vi "SMO.Basic--Process.vi"(8 "error in (no error)":errorcluster, 11 "SMO.Basic in":refnum<class "SMO.Basic.lvclass">) -> (0 "error out":errorcluster)   [LabVIEW 2013, in "SMO.Basic.lvclass"]
uses:
  SMO.Basic.lvclass
  <vilib>/JKI/JKI SMO/SMO/SMO.lvclass
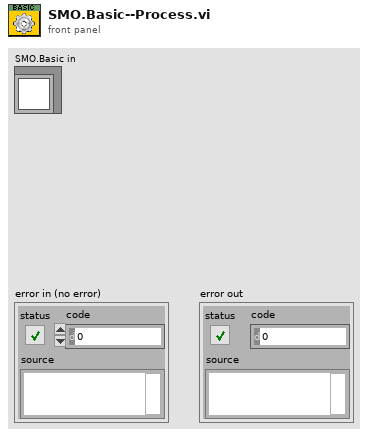
[diagram p1: front panel]
types:
  T1 = enum32{"invalid app kind", "Development System", "Run Time System", "Student Edition", "Embedded LabVIEW", "Evaluation", "Custom"}
  T2 = cluster{"Current VI Reference":refnum<vi>, "Close Panel on Exit?":bool, "error":errorcluster, "Standalone":bool}
  T3 = enum32{"Invalid", "Standard", "Closed", "Hidden", "Minimized", "Maximized"}
  T4 = typedef "SMO.lvclass/SMOState --Enum.ctl" = enum16{"unknown", "Created", "Started", "Stopped"}
  T5 = cluster{"Core":cluster{"Current VI Reference":refnum<vi>, "Close Panel on Exit?":bool, "error":errorcluster, "Standalone":bool}, "Self Reference":refnum<class "SMO.Basic.lvclass">, "Your string data":string}
  T6 = typedef "SMO.lvclass/Protected Events.ctl" = cluster{"StopProcesses":refnum<user-event>, "AbortProcesses":refnum<user-event>, "Config Changed":refnum<user-event>}
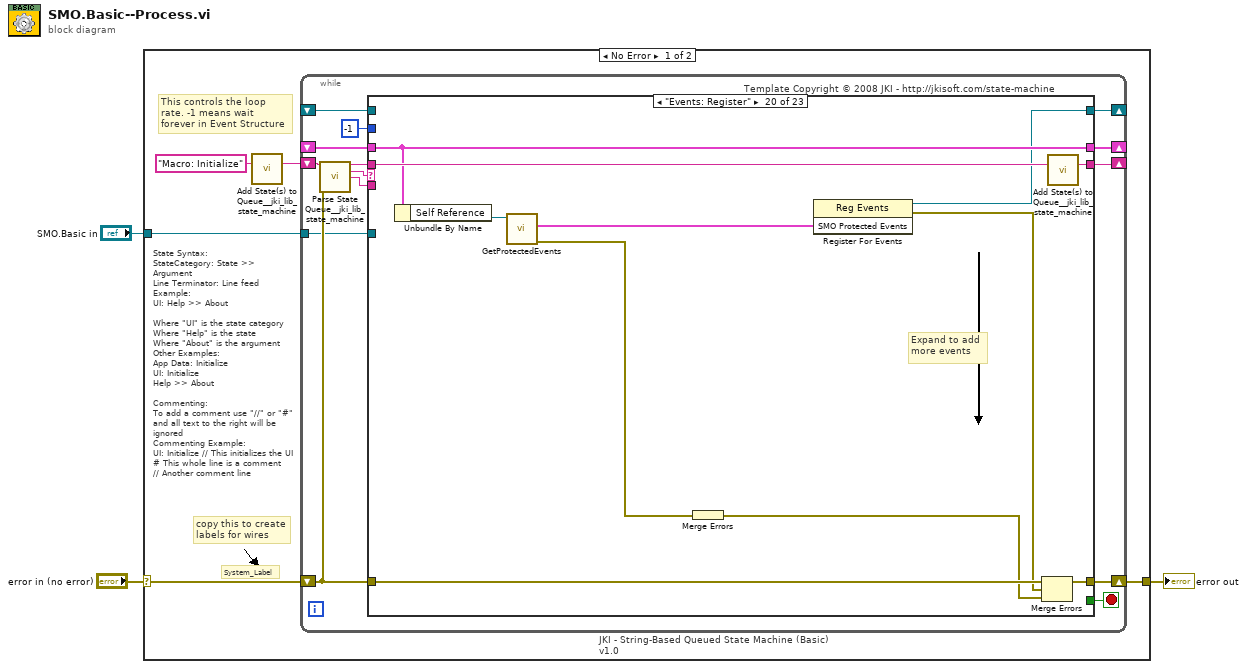
[diagram p0: block diagram]
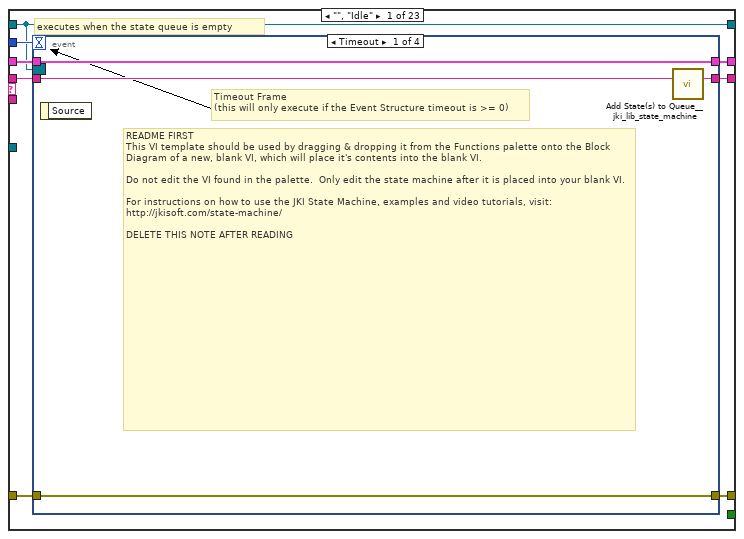
[diagram p2: hidden frame]
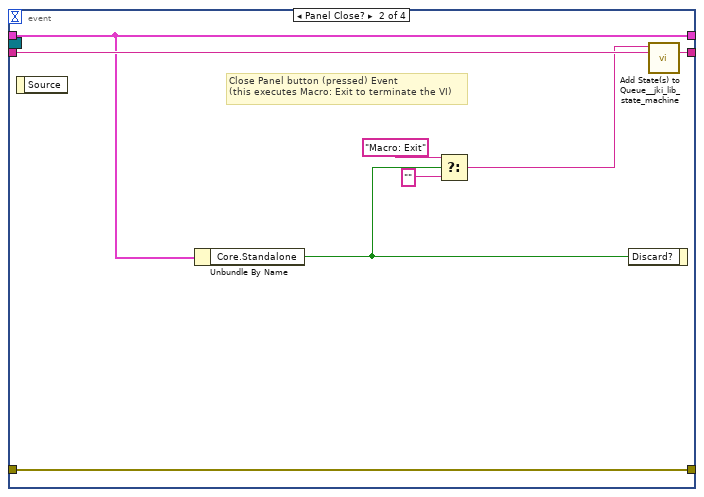
[diagram p3: hidden frame]
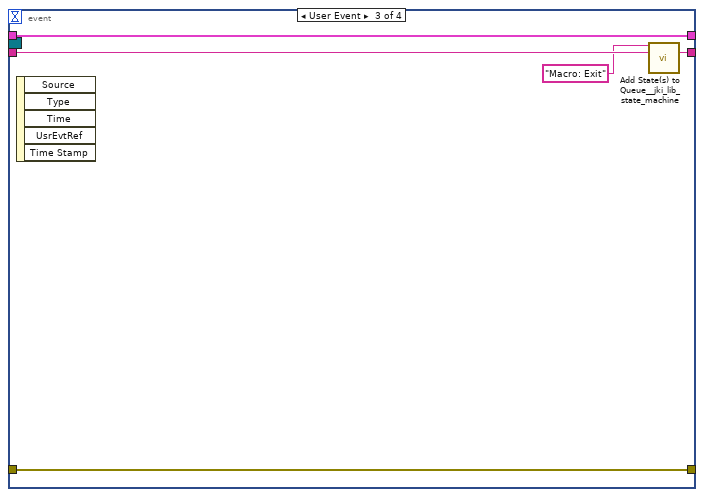
[diagram p4: hidden frame]
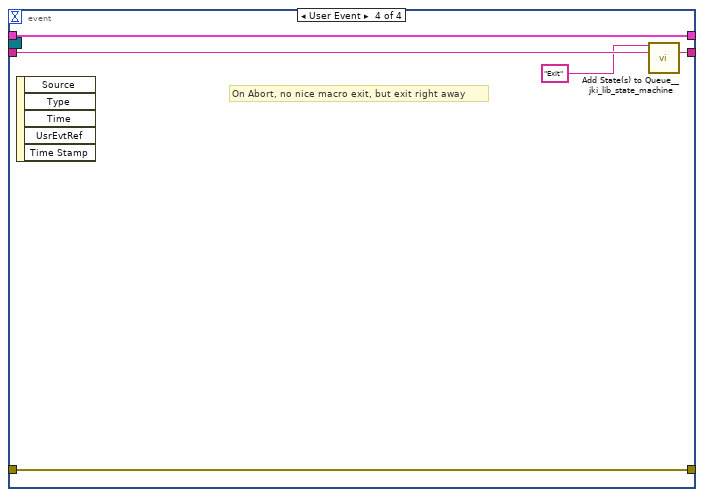
[diagram p5: hidden frame]
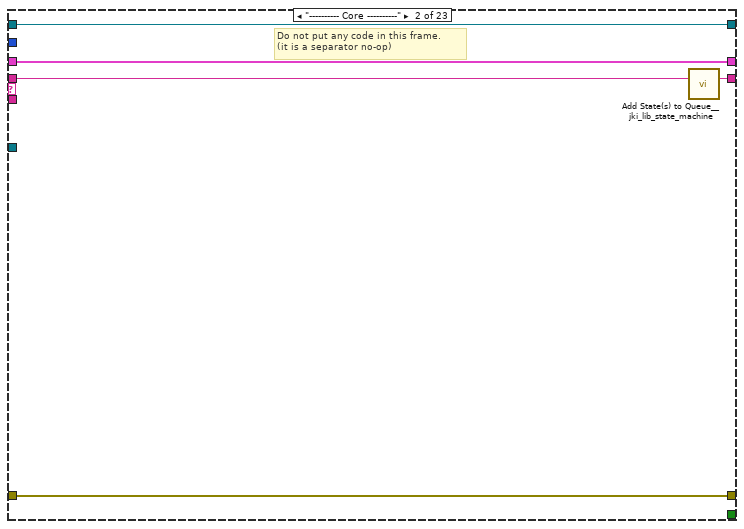
[diagram p6: hidden frame]
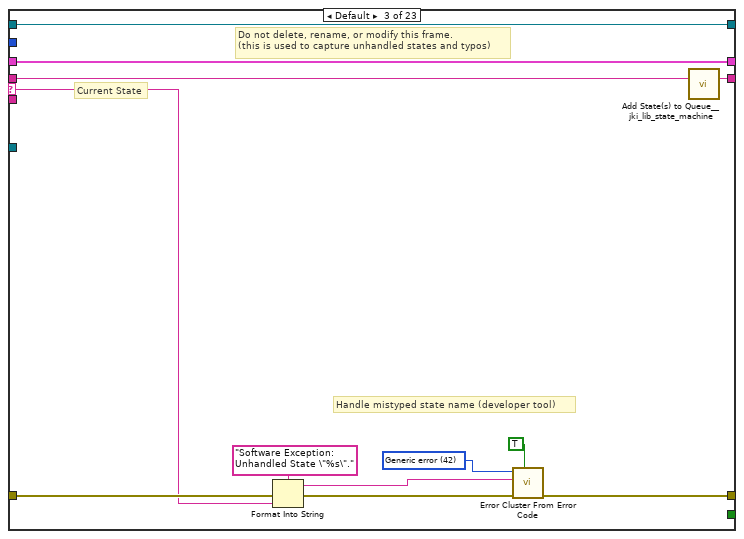
[diagram p7: hidden frame]
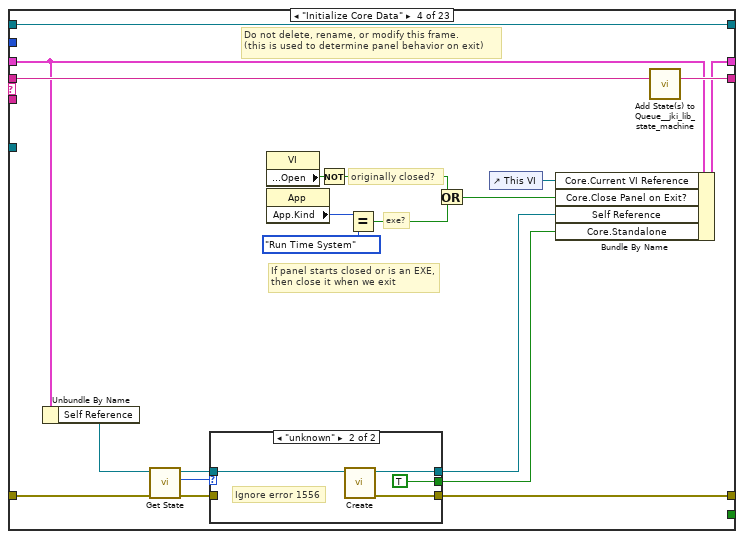
[diagram p8: hidden frame]
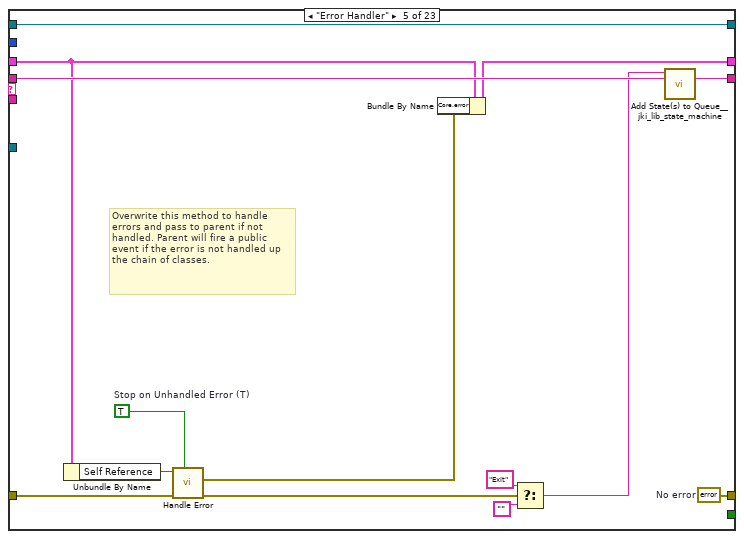
[diagram p10: hidden frame]
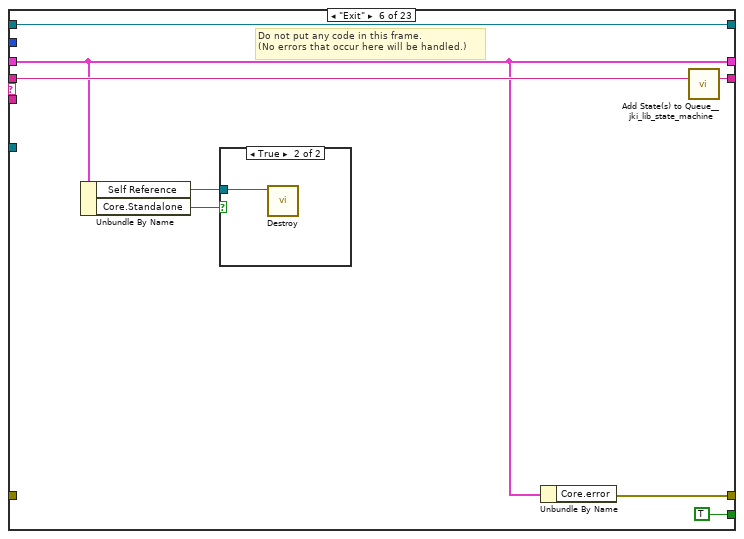
[diagram p11: hidden frame]
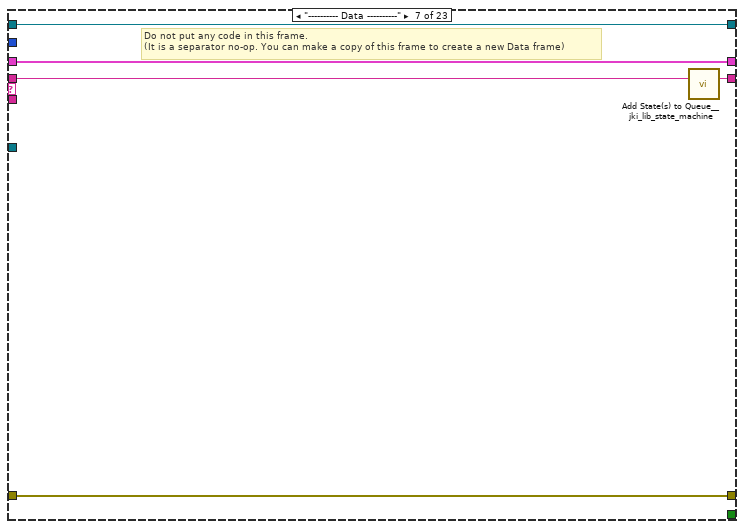
[diagram p13: hidden frame]
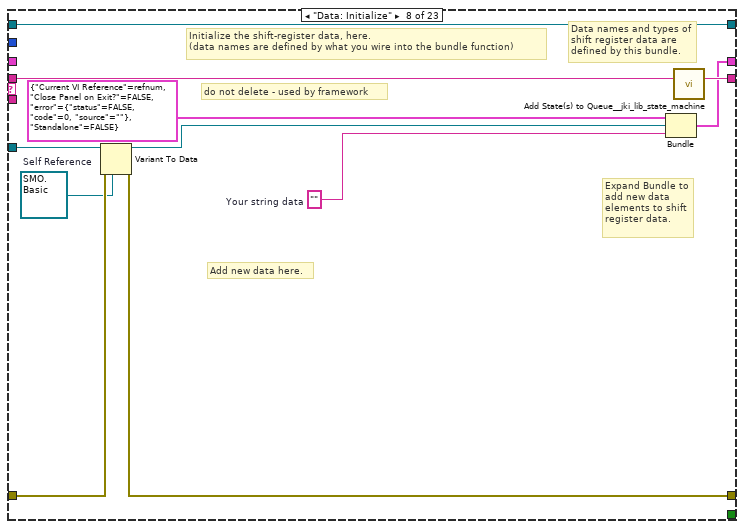
[diagram p14: hidden frame]
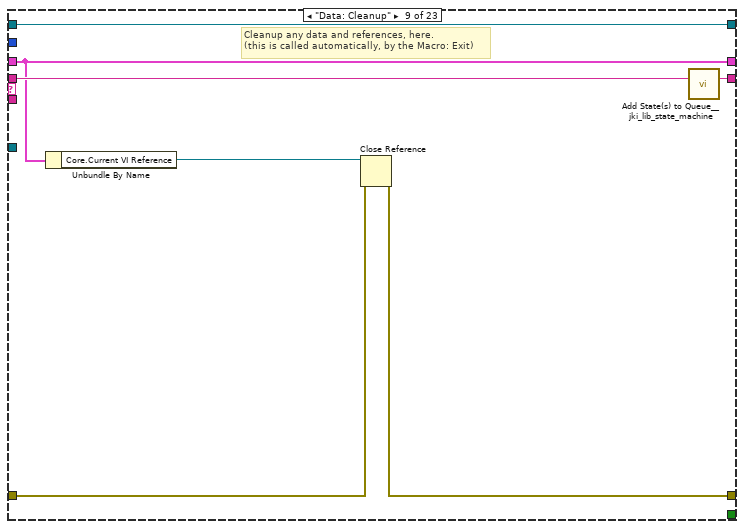
[diagram p15: hidden frame]
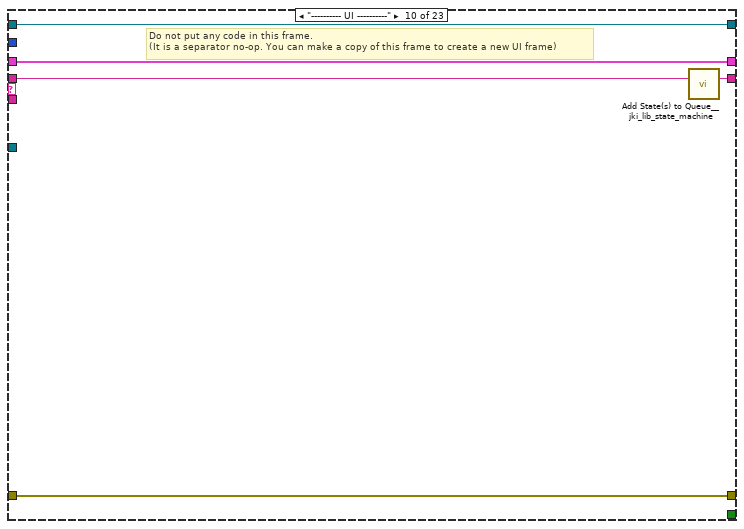
[diagram p16: hidden frame]
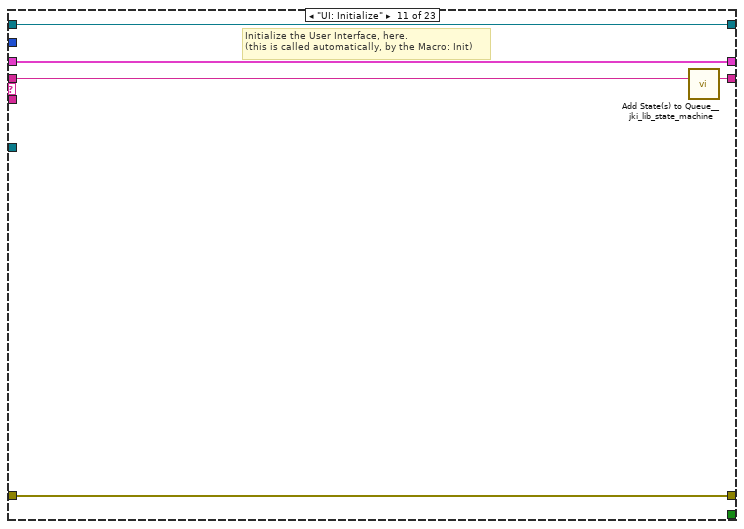
[diagram p17: hidden frame]
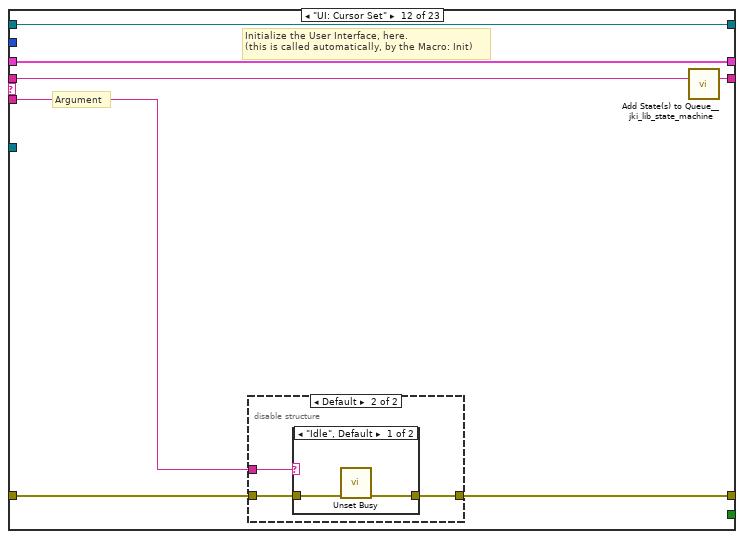
[diagram p18: hidden frame]
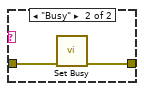
[diagram p20: hidden frame]
diagram:
  n1 = case shown="No Error" "error in (no error)" {
    selector: "error in (no error)" -> [w5 w280]
    tunnel: "SMO.Basic in" -> [w6 _]
    tunnel: [w4 w280] -> w3
    frame No Error {
      # "State Syntax:\nStateCategory: State >> Argument\nLine Terminator: Line feed\nExample:\nUI: Help >> About\n\nWhere \"UI\" is the state category\nWhere \"Help\" is the state\nWhere \"About\" is the argument\nOther Examples:\nApp Data: Initialize\nUI: Initialize\nHelp >> About\n\nCommenting:\nTo add a comment use \"//\" or \"#\" and all text to the right will be ignored\nCommenting Example:\nUI: Initialize // This initializes the UI\n# This whole line is a comment\n// Another comment line"
      # "copy this to create labels for wires"
      # "This controls the loop rate. -1 means wait forever in Event Structure"
      # "System_Label"
      n2 = call <vilib>:"Add State(s) to Queue__jki_lib_state_machine.vi"("State(s) in (\"\")"="Macro: Initialize") -> ("States Out"=w8:string)  [unwired: 14 in]
      n3 = while "JKI - String-Based Queued State Machine (Basic) v1.0" {
        shift-right: [w15] -> _
        shift-left: _ -> [w14]
        shift-right: [w18] -> w4
        shift-left: w5 -> [w12]
        shift-right: [w17] -> _
        shift-left: w8 -> [w19]
        tunnel: w6 -> [w11]
        shift-right: [w10] -> _
        shift-left: _ -> [w9]
        stop <- w16 stop-if-true
        # "Template Copyright © 2008 JKI - http://jkisoft.com/state-machine"
        n4 = call <vilib>:"Parse State Queue__jki_lib_state_machine.vi"("State Queue"=w19, "Error In (no error)"=w12) -> ("Remaining States"=w21:string, "Current State"=w22:string, "Arguments"=w20:string)  [unwired: 11 in]
        n5 = case shown="\"Events: Register\"" w22 {
          selector: w22 -> [_ _ w59 _ _ _ _ _ _ _ _ _ _ _ _ _ _ _ _ _ _ _ _]
          tunnel: w21 -> [w30 w57 w63 w89 w109 w117 w123 w134 w141 w146 w151 w158 w174 w206 w212 w223 w228 w237 w250 w261 w267 w272 w279]
          tunnel: w20 -> [_ _ _ _ _ _ _ _ _ _ _ w152 w168 _ _ _ _ _ _ _ _ _ _]
          tunnel: w14 -> [w28 w54 w61 w78 w103 w112 w120 _ w136 w143 w149 w156 w170 w203 w208 w214 w225 w234 w247 w259 w265 w270 w275]
          tunnel: [w27 w55 w65 w73 w104 w113 w121 w129 w137 w144 w148 w153 w171 w204 w210 w221 w226 w231 w248 w254 w263 w268 w276] -> w18
          tunnel: w12 -> [w26 w55 w64 w77 w105 _ w121 w130 w138 w144 w148 w154 w172 w204 w210 w221 w226 w232 w248 w255 w263 w268 w276]
          tunnel: [w29 w56 w62 w88 w108 w116 w122 w133 w140 w145 w150 w157 w173 w205 w211 w222 w227 w236 w249 w260 w266 w271 w278] -> w17
          tunnel: [_ _ _ _ _ TRUE _ _ _ _ _ _ _ _ _ _ _ _ _ _ _ _ _] -> w16
          tunnel: [w25 w54 w61 w87 w102 w112 w120 w132 w136 w143 w149 w156 w170 w203 w208 w214 w225 w234 w247 w259 w265 w270 w274] -> w15
          tunnel: -1 ("Timeout") -> [w24 _ _ _ _ _ _ _ _ _ _ _ _ _ _ _ _ _ _ _ _ _ _]
          tunnel: w11 -> [_ _ _ _ _ _ _ w127 _ _ _ _ _ _ _ _ _ _ _ _ _ _ _]
          tunnel: [w23 w53 w58 w80 w107 w114 w119 w125 w135 w142 w147 w155 w167 w202 w209 w215 w224 w235 w246 w258 w264 w269 w277] -> w10
          tunnel: w9 -> [w23 w53 w58 w80 w107 w114 w119 w125 w135 w142 w147 w155 w167 w202 w209 w215 w224 w235 w246 _ w264 w269 w277]
          frame "", "Idle" {
            # "executes when the state queue is empty"
            n6 = event shown="[0] Timeout" {
              selector: w23 -> [_ _ _ _]
              dyn-events: _ -> [_ _ _ _]
              timeout: w24 -> [_ _ _ _]
              tunnel: w30 -> [w34 w42 w47 w52]
              tunnel: [w33 w41 w46 w51] -> w29
              tunnel: w28 -> [w32 w39 w44 w49]
              tunnel: [w31 w40 w45 w50] -> w27
              tunnel: w26 -> [w31 w40 w45 w50]
              tunnel: [w32 w39 w44 w49] -> w25
              event Timeout {
                # "README FIRST\nThis VI template should be used by dragging & dropping it from the Functions palette onto the Block Diagram of a new, blank VI, which will place it's contents into the blank VI.\n\nDo not edit the VI found in the palette.  Only edit the state machine after it is placed into your blank VI.\n\nFor instructions on how to use the JKI State Machine, examples and video tutorials, visit:\nhttp://jkisoft.com/state-machine/\n\nDELETE THIS NOTE AFTER READING"
                # "Timeout Frame\n(this will only execute if the Event Structure timeout is >= 0)"
                n7 = event-data() -> ()  [unwired: 1 in, 1 out]
                n8 = call <vilib>:"Add State(s) to Queue__jki_lib_state_machine.vi"("State(s) in (\"\")"=w34) -> ("States Out"=w33:string)  [unwired: 14 in]
              }
              event Panel Close? {
                # "Close Panel button (pressed) Event\n(this executes Macro: Exit to terminate the VI)"
                n9 = event-data() -> ()  [unwired: 1 in, 1 out]
                n10 = Unbundle By Name(w39) -> ("Core.Standalone"=w38:bool)
                n11 = Select(t="Macro: Exit", s=w38, f="") -> (s? t:f=w35:string)
                n12 = event-data("Discard?"=w38) -> ()  [unwired: 1 in, 1 out]
                n13 = call <vilib>:"Add State(s) to Queue__jki_lib_state_machine.vi"("State(s) in Front (\"\")"=w35, "State(s) in (\"\")"=w42) -> ("States Out"=w41:string)  [unwired: 13 in]
              }
              event User Event {
                n14 = event-data() -> ()  [unwired: 1 in, 5 out]
                n15 = call <vilib>:"Add State(s) to Queue__jki_lib_state_machine.vi"("State(s) in Front (\"\")"="Macro: Exit", "State(s) in (\"\")"=w47) -> ("States Out"=w46:string)  [unwired: 13 in]
              }
              event User Event {
                # "On Abort, no nice macro exit, but exit right away"
                n16 = event-data() -> ()  [unwired: 1 in, 5 out]
                n17 = call <vilib>:"Add State(s) to Queue__jki_lib_state_machine.vi"("State(s) in Front (\"\")"="Exit", "State(s) in (\"\")"=w52) -> ("States Out"=w51:string)  [unwired: 13 in]
              }
            }
          }
          frame "---------- Core ----------" {
            # "Do not put any code in this frame.\n(it is a separator no-op)"
            n18 = call <vilib>:"Add State(s) to Queue__jki_lib_state_machine.vi"("State(s) in (\"\")"=w57) -> ("States Out"=w56:string)  [unwired: 14 in]
          }
          frame Default {
            w68 = 42 items=["No error", "Argument error", "Memory is full", "Out of zone", "End of file", "File already open", "Generic file I/O error", "File not found", "File permission error", "Disk is full", "Duplicate path", "Too many files open", "System feature not enabled", "Resource file not found", "Cannot add resource", "Resource not found", "Image not found", "Image memory error", "Pen does not exist", "Config type invalid", "Config token not found", "Config parse error", "Config memory error", "Bad external code format", "Bad external code offset", "External code not present", "Null window", "Destroy window error", "Null menu", "Print aborted", "Bad print record", "Print driver error", "Windows error during printing", "Memory error during printing", "Print dialog error", "Generic print error", "Invalid device refnum", "Device not found", "Device parameter error", "Device unit error", "Cannot open device", "Device call aborted", "Generic error", "Cancelled by user", "Object ID too low", "Object ID too high", "Object not in heap", "Unknown heap", "Unknown object (invalid DefProc)", "Unknown object (DefProc not in table)", "Message out of range", "Invalid (null) method", "Unknown message", "Manager call not supported", "Bad address", "Network operation in progress", "Network operation timed out", "Connection is busy", "Network attribute not supported", "Network error", "Address in use", "System out of memory", "Connection aborted", "Connection refused", "Not connected", "Already connected", "Connection closed", "Initialization error (interapplication manager)", "Bad occurrence", "Wait on unbound occurrence handler", "Occurrence queue overflow", "Datalog type conflict", "Unused", "Unrecognized type (interapplication manager)", "Memory corrupt", "Failed to make temporary DLL", "Old CIN version", "Drag socket not found", "Failed to load drop-object", "Failed to register OLE object", "Failed to release OLE object", "Format specifier type mismatch", "Unknown format specifier", "Too few format specifiers", "Too many format specifiers", "Scan failed", "Newer CIN version", "Error converting to variant", "Runtime menu error", "Password tampered", "Variant attribute not found", "Incompatible variant data type", "Event data is not available", "Event Store is not present", "Occurrence is not found", "Event Queue is not created", "Event info is not available", "Refnum passed is NULL", "Error retrieving Class GUID", "Error retrieving CoClass GUID", "Error retrieving TypeLib GUID.", "Bad built application magic bytes.", "Specific driver is different from the specific driver associated with the Logical Name.", "There is no session opened to the class driver.", "Max Error", "MAX - Error with config objects", "MAX - Error loading configuration", "MAX - Group not supported"]
            # "Current State"
            # "Do not delete, rename, or modify this frame.\n(this is used to capture unhandled states and typos)"
            # "Handle mistyped state name (developer tool)"
            n19 = Format Into String(format string="Software Exception: Unhandled State \"%s\"." ("message"), error in=w64, w59) -> (resulting string=w67:string, error out=w66:errorcluster)  [unwired: 1 in]
            n20 = call <vilib>:"Error Cluster From Error Code.vi"("show call chain? (False)"=TRUE, "error in (no error)"=w66, "error message (\"\")"=w67, "error code (0)"=w68) -> ("error out"=w65:errorcluster)  [unwired: 5 in]
            n21 = call <vilib>:"Add State(s) to Queue__jki_lib_state_machine.vi"("State(s) in (\"\")"=w63) -> ("States Out"=w62:string)  [unwired: 14 in]
          }
          frame "Initialize Core Data" {
            # "Do not delete, rename, or modify this frame.\n(this is used to determine panel behavior on exit)"
            # "originally closed?"
            # "exe?"
            # "If panel starts closed or is an EXE, then close it when we exit"
            n22 = Unbundle By Name(w78) -> ("Self Reference"=w76:refnum<class "SMO.Basic.lvclass">)
            n23 = call <vilib>:"Get State.vi"("error in (no error)"=w77, "SMO"=w76) -> ("error out"=w74:errorcluster, "SMO State"=w70:T4, "SMO out"=w75:refnum<class "SMO.Basic.lvclass">)  [unwired: 7 in]
            n24 = case shown="\"unknown\"" w70 {
              tunnel: w75 -> [w91 w95]
              tunnel: w74 -> [w90 _]
              tunnel: [w90 w94] -> w73
              tunnel: [w91 w93] -> w72
              tunnel: [_ TRUE] -> w71
              frame Default {
              }
              frame "unknown" {
                # "Ignore error 1556"
                n25 = call <vilib>:"Create.vi"("SMO"=w95) -> ("error out"=w94:errorcluster, "SMO out"=w93:refnum<class "SMO.Basic.lvclass">)  [unwired: 8 in, 1 out]
              }
            }
            n26 = property class="VI"() -> ("Front Panel.Open"=w86:bool)  [unwired: 2 in, 2 out]
            n27 = property class="App"() -> ("App.Kind"=w85:T1)  [unwired: 2 in, 2 out]
            n28 = Not(x=w86) -> (.not. x?=w83:bool)
            n29 = Equal?(x=w85, y=T1."Run Time System" ("Application:Kind")) -> (x = y?=w82:bool)
            n30 = Or(x=w83, y=w82) -> (x .or. y?=w81:bool)
            n31 = control-ref of="This VI"() -> (w79:refnum<vi>)
            n32 = Bundle By Name(cluster=w78, "Core.Current VI Reference"=w79, "Core.Close Panel on Exit?"=w81, "Self Reference"=w72, "Core.Standalone"=w71) -> (w87:T5)
            n33 = call <vilib>:"Add State(s) to Queue__jki_lib_state_machine.vi"("State(s) in (\"\")"=w89) -> ("States Out"=w88:string)  [unwired: 14 in]
          }
          frame "Error Handler" {
            w96 = TRUE  # Stop on Unhandled Error (T)
            w104 = errorcluster {"status"=FALSE, "code"=0, "source"=""}  # No error
            # "Overwrite this method to handle errors and pass to parent if not handled. Parent will fire a public event if the error is not handled up the chain of classes."
            n34 = Unbundle By Name(w103) -> ("Self Reference"=w106:refnum<class "SMO.Basic.lvclass">)
            n35 = call-dynamic "Handle Error.vi"("Stop on Unhandled Error (T)"=w96, "error in"=w105, "SMO"=w106) -> ("handling error"=w97:errorcluster, "Unhandled error"=w100:errorcluster)  [unwired: 6 in, 1 out]
            n36 = Bundle By Name(cluster=w103, "Core.error"=w100) -> (w102:T5)
            n37 = Select(t="Exit", s=w97, f="") -> (s? t:f=w101:string)
            n38 = call <vilib>:"Add State(s) to Queue__jki_lib_state_machine.vi"("State(s) in Front (\"\")"=w101, "State(s) in (\"\")"=w109) -> ("States Out"=w108:string)  [unwired: 13 in]
          }
          frame "Exit" {
            # "Do not put any code in this frame.\n(No errors that occur here will be handled.)"
            n39 = Unbundle By Name(w112) -> ("Self Reference"=w111:refnum<class "SMO.Basic.lvclass">, "Core.Standalone"=w110:bool)
            n40 = case shown="True" w110 {
              tunnel: w111 -> [_ w118]
              frame False {
              }
              frame True {
                n41 = call <vilib>:"Destroy.vi"("SMO"=w118) -> ()  [unwired: 10 in, 1 out]
              }
            }
            n42 = Unbundle By Name(w112) -> ("Core.error"=w113:errorcluster)
            n43 = call <vilib>:"Add State(s) to Queue__jki_lib_state_machine.vi"("State(s) in (\"\")"=w117) -> ("States Out"=w116:string)  [unwired: 14 in]
          }
          frame "---------- Data ----------" {
            # "Do not put any code in this frame.\n(It is a separator no-op. You can make a copy of this frame to create a new Data frame)"
            n44 = call <vilib>:"Add State(s) to Queue__jki_lib_state_machine.vi"("State(s) in (\"\")"=w123) -> ("States Out"=w122:string)  [unwired: 14 in]
          }
          frame "Data: Initialize" {
            w128 = refnum<class "SMO.Basic.lvclass"> refnum  # Self Reference
            w131 = ""  # Your string data
            # "do not delete - used by framework"
            # "Expand Bundle to add new data elements to shift register data."
            # "Add new data here."
            # "Data names and types of shift register data are defined by this bundle."
            # "Initialize the shift-register data, here.\n(data names are defined by what you wire into the bundle function)"
            n45 = Variant To Data(error in=w130, type=w128, Variant=w127) -> (data=w126:refnum<class "SMO.Basic.lvclass">, error out=w129:errorcluster)
            n46 = Bundle("Core"=T2 {"Current VI Reference"=refnum, "Close Panel on Exit?"=FALSE, "error"={"status"=FALSE, "code"=0, "source"=""}, "Standalone"=FALSE}, "Self Reference"=w126, "Your string data"=w131) -> (w132:T5)  [unwired: 1 in]
            n47 = call <vilib>:"Add State(s) to Queue__jki_lib_state_machine.vi"("State(s) in (\"\")"=w134) -> ("States Out"=w133:string)  [unwired: 14 in]
          }
          frame "Data: Cleanup" {
            # "Cleanup any data and references, here.\n(this is called automatically, by the Macro: Exit)"
            n48 = Unbundle By Name(w136) -> ("Core.Current VI Reference"=w139:refnum<vi>)
            n49 = Close Reference(reference=w139, error in (no error)=w138) -> (error out=w137:errorcluster)
            n50 = call <vilib>:"Add State(s) to Queue__jki_lib_state_machine.vi"("State(s) in (\"\")"=w141) -> ("States Out"=w140:string)  [unwired: 14 in]
          }
          frame "---------- UI ----------" {
            # "Do not put any code in this frame.\n(It is a separator no-op. You can make a copy of this frame to create a new UI frame)"
            n51 = call <vilib>:"Add State(s) to Queue__jki_lib_state_machine.vi"("State(s) in (\"\")"=w146) -> ("States Out"=w145:string)  [unwired: 14 in]
          }
          frame "UI: Initialize" {
            # "Initialize the User Interface, here.\n(this is called automatically, by the Macro: Init)"
            n52 = call <vilib>:"Add State(s) to Queue__jki_lib_state_machine.vi"("State(s) in (\"\")"=w151) -> ("States Out"=w150:string)  [unwired: 14 in]
          }
          frame "UI: Cursor Set" {
            # "Argument"
            # "Initialize the User Interface, here.\n(this is called automatically, by the Macro: Init)"
            n53 = disable-structure shown="Default" {
              disable-tunnel: w154 -> [w159 w162]
              disable-tunnel: [w159 w161] -> w153
              disable-tunnel: w152 -> [_ w160]
              frame condition #0 {
              }
              frame condition #1 (active) {
                n54 = case shown="\"Idle\", Default" w160 {
                  tunnel: w162 -> [w164 w166]
                  tunnel: [w163 w165] -> w161
                  frame "Idle", Default {
                    n55 = call <vilib>:"Unset Busy.vi"("error in (no error)"=w164) -> ("error out"=w163:errorcluster)  [unwired: 10 in]
                  }
                  frame "Busy" {
                    n56 = call <vilib>:"Set Busy.vi"("error in (no error)"=w166) -> ("error out"=w165:errorcluster)  [unwired: 9 in, 1 out]
                  }
                }
              }
            }
            n57 = call <vilib>:"Add State(s) to Queue__jki_lib_state_machine.vi"("State(s) in (\"\")"=w158) -> ("States Out"=w157:string)  [unwired: 14 in]
          }
          frame "UI: Front Panel State" {
            # "Argument"
            # "Set Front Panel Open or Closed\n(Usage: \"UI: Front Panel State >> Open|Close\")"
            n58 = Unbundle By Name(w170) -> ("Core.Current VI Reference"=w169:refnum<vi>)
            n59 = disable-structure shown="Default" {
              disable-tunnel: w172 -> [w178 w201]
              disable-tunnel: [w177 w201] -> w171
              disable-tunnel: w169 -> [w176 _]
              disable-tunnel: w168 -> [w175 _]
              frame condition #0 (active) {
                n60 = case shown="\"Close\"" w175 {
                  tunnel: w178 -> [w182 w195]
                  tunnel: [w184 w196] -> w177
                  tunnel: w176 -> [w183 w193]
                  frame "Open", Default {
                    n61 = property class="VI"(reference=w183, error in=w182) -> (reference out=w180:refnum<vi>, error out=w181:errorcluster, "FP.State"=w179:T3)
                    n62 = case shown="\"Closed\"" w179 {
                      tunnel: [w187 w190] -> w184
                      tunnel: w181 -> [w186 w190]
                      tunnel: w180 -> [w185 _]
                      frame "Closed" {
                        n63 = invoke class="VI" method="FP.Open"(reference=w185, error in=w186, "Activate"=TRUE, "State"=T3."Standard") -> (error out=w187:errorcluster)  [unwired: 1 in, 4 out]
                      }
                      frame Default {
                      }
                    }
                  }
                  frame "Close" {
                    n64 = property class="VI"(reference=w193, error in=w195) -> (reference out=w192:refnum<vi>, error out=w194:errorcluster, "FP.State"=w191:T3)
                    n65 = case shown="Default" w191 {
                      tunnel: [w197 w200] -> w196
                      tunnel: w194 -> [w197 w199]
                      tunnel: w192 -> [_ w198]
                      frame "Invalid", "Closed" {
                      }
                      frame Default {
                        n66 = invoke class="VI" method="FP.Close"(reference=w198, error in=w199) -> (error out=w200:errorcluster)  [unwired: 1 in, 2 out]
                      }
                    }
                  }
                }
              }
              frame condition #1 {
              }
            }
            n67 = call <vilib>:"Add State(s) to Queue__jki_lib_state_machine.vi"("State(s) in (\"\")"=w174) -> ("States Out"=w173:string)  [unwired: 14 in]
          }
          frame "---------- Macro ----------" {
            # "Do not put any code in this frame.\n(It is a separator no-op. You can make a copy of this frame to create a new Macro frame)"
            n68 = call <vilib>:"Add State(s) to Queue__jki_lib_state_machine.vi"("State(s) in (\"\")"=w206) -> ("States Out"=w205:string)  [unwired: 14 in]
          }
          frame "Macro: Initialize" {
            # "Initialization Macro\n(This is called once, when the VI starts)"
            n69 = call <vilib>:"Add State(s) to Queue__jki_lib_state_machine.vi"("State(s) in Front (\"\")"="Data: Initialize\nInitialize Core Data\nEvents: Register\nProcess: Sync", "State(s) in (\"\")"=w212) -> ("States Out"=w211:string)  [unwired: 13 in]
          }
          frame "Macro: Exit" {
            # "Exit Macro\n(This is called once, when the VI exits)"
            n70 = Unbundle By Name(w214) -> ("Core.Close Panel on Exit?"=w220:bool)
            n71 = Select(t="UI: Front Panel State >> Close", s=w220, f="") -> (s? t:f=w217:string)
            n72 = call <vilib>:"Add State(s) to Queue__jki_lib_state_machine.vi"("State(s) in (\"\")"=w217, "State(s) at Back (\"\")"="Data: Cleanup\nEvents: Unregister\nProcess: Sync\nExit") -> ("States Out"=w216:string)  [unwired: 13 in]
            n73 = call <vilib>:"Add State(s) to Queue__jki_lib_state_machine.vi"("State(s) in Front (\"\")"=w216, "State(s) in (\"\")"=w223) -> ("States Out"=w222:string)  [unwired: 13 in]
          }
          frame "---------- Process ----------" {
            # "Template Separator\n(You can make a copy of, or modify, this frame)"
            n74 = call <vilib>:"Add State(s) to Queue__jki_lib_state_machine.vi"("State(s) in (\"\")"=w228) -> ("States Out"=w227:string)  [unwired: 14 in]
          }
          frame "Process: Sync" {
            n75 = Unbundle By Name(w234) -> ("Self Reference"=w233:refnum<class "SMO.Basic.lvclass">, "Core.Standalone"=w229:bool)
            n76 = case shown="False" w229 {
              tunnel: w233 -> [w241 _]
              tunnel: w232 -> [w240 w245]
              tunnel: [w239 w245] -> w231
              tunnel: [w238 _] -> w230
              frame False {
                n77 = call <vilib>:"WaitOnProcessSync.vi"("error in (no error)"=w240, "SMO"=w241) -> ("error out"=w239:errorcluster, "Don't run?"=w244:bool)  [unwired: 7 in, 1 out]
                n78 = Select(t="Data: Cleanup\nEvents: Unregister\nExit", s=w244, f="") -> (s? t:f=w238:string)
              }
              frame True {
              }
            }
            n79 = call <vilib>:"Add State(s) to Queue__jki_lib_state_machine.vi"("State(s) in Front (\"\")"=w230, "State(s) in (\"\")"=w237) -> ("States Out"=w236:string)  [unwired: 13 in]
          }
          frame "---------- Events ----------" {
            # "Template Separator\n(You can make a copy of, or modify, this frame)"
            n80 = call <vilib>:"Add State(s) to Queue__jki_lib_state_machine.vi"("State(s) in (\"\")"=w250) -> ("States Out"=w249:string)  [unwired: 14 in]
          }
          frame "Events: Register" {
            # "Expand to add\nmore events"
            n81 = Unbundle By Name(w259) -> ("Self Reference"=w256:refnum<class "SMO.Basic.lvclass">)
            n82 = call <vilib>:"GetProtectedEvents.vi"("SMO"=w256) -> ("error out"=w252:errorcluster, "SMO Protected Events"=w257:T6)  [unwired: 8 in, 1 out]
            n83 = Merge Errors(w252) -> (w251:errorcluster)
            n84 = register-events(w257) -> (reference out=w258:refnum<event-registration>, error out=w253:errorcluster)  [unwired: 2 in]
            n85 = Merge Errors(w255, w253, w251) -> (w254:errorcluster)
            n86 = call <vilib>:"Add State(s) to Queue__jki_lib_state_machine.vi"("State(s) in (\"\")"=w261) -> ("States Out"=w260:string)  [unwired: 14 in]
          }
          frame "Events: Unregister" {
            n87 = Unregister For Events(event registration refnum=w264, error in=w263) -> (error out=w262:errorcluster)
            n88 = call <vilib>:"Clear Errors.vi"("error in (no error)"=w262) -> ()  [unwired: 6 in, 1 out]
            n89 = call <vilib>:"Add State(s) to Queue__jki_lib_state_machine.vi"("State(s) in (\"\")"=w267) -> ("States Out"=w266:string)  [unwired: 14 in]
          }
          frame "---------- Action ----------" {
            n90 = call <vilib>:"Add State(s) to Queue__jki_lib_state_machine.vi"("State(s) in (\"\")"=w272) -> ("States Out"=w271:string)  [unwired: 14 in]
          }
          frame "Action: Template" {
            n91 = Unbundle By Name(w275) -> ("Self Reference"=w273:refnum<class "SMO.Basic.lvclass">)
            n92 = Bundle By Name(cluster=w275, "Self Reference"=w273) -> (w274:T5)
            n93 = call <vilib>:"Add State(s) to Queue__jki_lib_state_machine.vi"("State(s) in (\"\")"=w279) -> ("States Out"=w278:string)  [unwired: 14 in]
          }
        }
      }
    }
    frame Error {
    }
  }
  "error out" <- w3
